vi "Connect.vi"(8 "error in (no error)":errorcluster, 11 "TCP Comm":T1) -> (0 "error out":errorcluster)   [LabVIEW 2020, in "TCP Comms.lvlib"]
uses:
  TCP Comms.lvlib
  TCP Comm.ctl
  Ref Data.ctl
  State.ctl
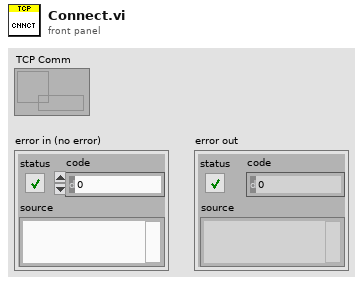
[diagram p1: front panel]
types:
  T1 = typedef "TCP Comms.lvlib/TCP Comm.ctl" = refnum<data-value>
  T2 = typedef "TCP Comms.lvlib/Ref Data.ctl" = cluster{"TCP":refnum<k5>, "State":T3, "Server":bool, "Host":string, "Port":u16, "Listener":refnum<k5>, "Start":bool, "Disconnect":bool, "TCP Valid":bool, "TLS Enabled":bool, "Immutable TLS":refnum<k36>, "Certificate DN":string}
  T3 = typedef "TCP Comms.lvlib/State.ctl" = enum16{"Idle", "Starting", "Connecting", "Connected", "Disconnecting", "Stopped"}
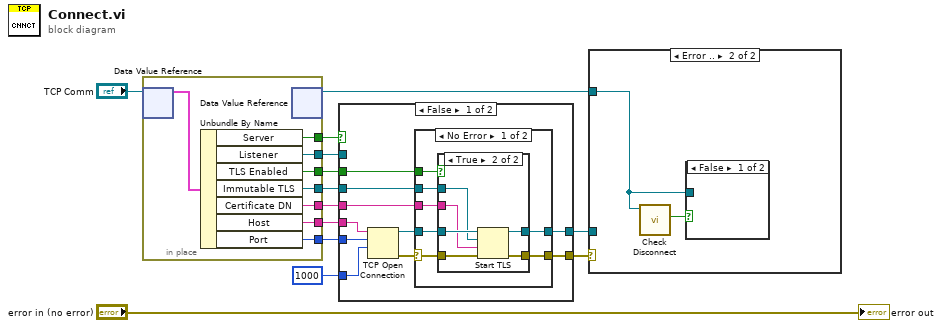
[diagram p0: block diagram]
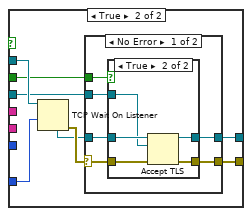
[diagram p4: hidden frame]
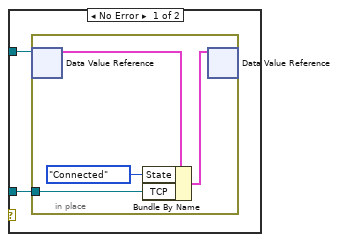
[diagram p7: hidden frame]
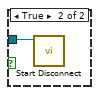
[diagram p8: hidden frame]
diagram:
  n1 = in-place {
    in-place-border: [w20] -> w11
    in-place-border: [w19] -> w12
    in-place-border: [w18] -> w5
    in-place-border: [w17] -> w4
    in-place-border: [w16] -> w3
    in-place-border: [w15] -> w2
    in-place-border: [w14] -> w1
    n2 = in-place-dvr #1("TCP Comm") -> (w21:T2)  [unwired: 1 out]
    n3 = Unbundle By Name(w21) -> ("Server"=w15:bool, "Listener"=w14:refnum<k5>, "TLS Enabled"=w17:bool, "Immutable TLS"=w18:refnum<k36>, "Certificate DN"=w16:string, "Host"=w20:string, "Port"=w19:u16)
    n4 = in-place-dvr #1() -> (w7:T1)  [unwired: 1 in, 1 out]
  }
  n5 = case shown="False" w2 {
    tunnel: w12 -> [w30 _]
    tunnel: w11 -> [w31 _]
    tunnel: [w24 w48] -> w9
    tunnel: [w22 w49] -> w8
    tunnel: 1000 ("timeout ms (wait forever: -1)") -> [w29 w55]
    tunnel: w5 -> [w25 w52]
    tunnel: w4 -> [w26 w53]
    tunnel: w3 -> [w23 _]
    tunnel: w1 -> [_ w54]
    frame False {
      n6 = TCP Open Connection(address=w31, remote port or service name=w30, timeout ms (60000)=w29) -> (connection ID=w27:refnum<k5>, error out=w28:errorcluster)  [unwired: 2 in]
      n7 = case shown="No Error" w28 {
        selector: w28 -> [w38 w47]
        tunnel: w27 -> [w37 _]
        tunnel: w26 -> [w35 _]
        tunnel: w25 -> [w34 _]
        tunnel: [w32 w47] -> w24
        tunnel: w23 -> [w36 _]
        tunnel: [w33 _] -> w22
        frame No Error {
          n8 = case shown="True" w35 {
            tunnel: w38 -> [w39 w46]
            tunnel: w37 -> [w40 w45]
            tunnel: w36 -> [_ w44]
            tunnel: w34 -> [_ w43]
            tunnel: [w40 w42] -> w33
            tunnel: [w39 w41] -> w32
            frame False {
            }
            frame True {
              n9 = Start TLS(8:w46, 9:w44, 10:w43, 11:w45) -> (0:w41:errorcluster, 3:w42:refnum<k5>)  [unwired: 2 in, 1 out]
            }
          }
        }
        frame Error {
        }
      }
    }
    frame True {
      n10 = TCP Wait On Listener(9:w55, 11:w54) -> (0:w51:errorcluster, 4:w50:refnum<k5>)  [unwired: 2 in, 3 out]
      n11 = case shown="No Error" w51 {
        selector: w51 -> [w61 w69]
        tunnel: w50 -> [w60 _]
        tunnel: w53 -> [w59 _]
        tunnel: w52 -> [w58 _]
        tunnel: [w56 w69] -> w48
        tunnel: [w57 _] -> w49
        frame No Error {
          n12 = case shown="True" w59 {
            tunnel: w61 -> [w62 w68]
            tunnel: w60 -> [w63 w67]
            tunnel: w58 -> [_ w66]
            tunnel: [w63 w65] -> w57
            tunnel: [w62 w64] -> w56
            frame False {
            }
            frame True {
              n13 = Accept TLS(8:w68, 10:w66, 11:w67) -> (0:w64:errorcluster, 3:w65:refnum<k5>)  [unwired: 1 in, 1 out]
            }
          }
        }
        frame Error {
        }
      }
    }
  }
  n14 = case shown="Error .." w9 {
    tunnel: w8 -> [w70 _]
    tunnel: w7 -> [w71 w76]
    frame No Error {
      n15 = in-place {
        in-place-border: w70 -> [w73]
        n16 = in-place-dvr #2(w71) -> (w75:T2)  [unwired: 1 out]
        n17 = Bundle By Name(cluster=w75, "State"=State."Connected", "TCP"=w73) -> (w74:T2)
        n18 = in-place-dvr #2(w74) -> ()  [unwired: 2 out]
      }
    }
    frame Error {
      n19 = call "Check Disconnect.vi"("TCP Comm"=w76) -> ("Disconnecting?"=w77:bool)  [unwired: 9 in, 1 out]
      n20 = case shown="False" w77 {
        tunnel: w76 -> [_ w78]
        frame False {
        }
        frame True {
          n21 = call "Start Disconnect.vi"("TCP Comm"=w78) -> ()  [unwired: 10 in, 1 out]
        }
      }
    }
  }
  "error out" <- "error in (no error)"
